vi "enable or disable module.vi"(6 "source":string, 7 "timeout":i32, 8 "error in (no error)":errorcluster, 9 "request type":T1, 10 "Module ID":string, 11 "Standard Engine Runtime in":refnum<class "Standard Engine Runtime.lvclass">) -> (0 "error out":errorcluster, 3 "Standard Engine Runtime out":refnum<class "Standard Engine Runtime.lvclass">)   [LabVIEW 2013, in "Standard Engine Runtime.lvclass"]
uses:
  Standard Engine Runtime.lvclass
  main engine/message request type.ctl
  main engine/message to engine.ctl
  global counter.vi
  main engine/main engine.lvlib
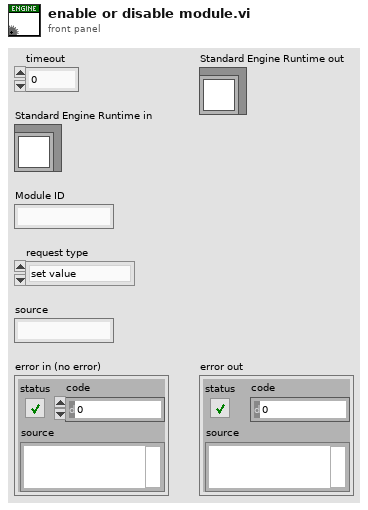
[diagram p1: front panel]
types:
  T1 = typedef "main engine.lvlib/message request type.ctl" = enum8{"set value", "disable module", "enable module"}
  T2 = typedef "main engine.lvlib/message to engine.ctl" = cluster{"request type":T1, "message ID":u8, "message field 1":u64, "message field 2":u64, "message field 3":u64, "message field 4":u64}
  T3 = typedef "main engine.lvlib/message from engine.ctl" = cluster{"response type":T4, "message ID":u8, "error code":i32}
  T4 = typedef "main engine.lvlib/message response type.ctl" = enum8{"ok", "error"}
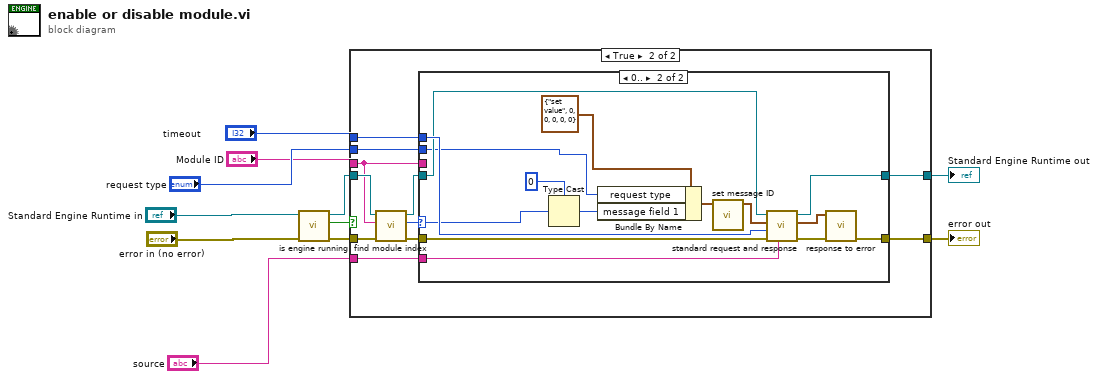
[diagram p0: block diagram]
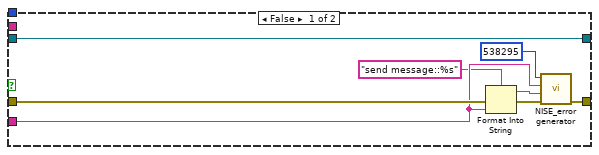
[diagram p2: hidden frame]
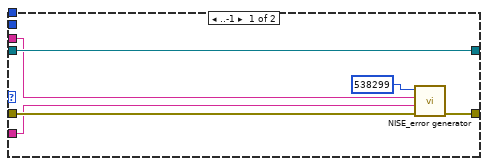
[diagram p3: hidden frame]
diagram:
  n1 = call "is engine running.vi"("error in"="error in (no error)", "Standard Engine Runtime in"="Standard Engine Runtime in") -> ("error out"=w7:errorcluster, "running?"=w3:bool, "Standard Engine Runtime out"=w5:refnum<class "Standard Engine Runtime.lvclass">)  [unwired: 7 in]
  n2 = case shown="True" w3 {
    tunnel: [w19 w30] -> w4
    tunnel: w5 -> [w19 w24]
    tunnel: [w17 w27] -> w6
    tunnel: w7 -> [w18 w26]
    tunnel: "timeout" -> [_ w28]
    tunnel: "source" -> [w14 w29]
    tunnel: "Module ID" -> [_ w21]
    tunnel: "request type" -> [_ w20]
    frame False {
      n3 = Format Into String(format string="send message::%s" ("source"), error in=w18, w14) -> (resulting string=w15:string, error out=w16:errorcluster)  [unwired: 1 in]
      n4 = call <vilib>:"NISE_error generator.vi"("error in"=w16, "source"=w15, "append error message"=w14, "error code (0)"=538295) -> ("error out"=w17:errorcluster)  [unwired: 5 in]
    }
    frame True {
      n5 = call "find module index.vi"("error in"=w26, "module ID"=w21, "Standard Engine Runtime in"=w24) -> ("error out"=w25:errorcluster, "index"=w22:i32, "Standard Engine Runtime out"=w23:refnum<class "Standard Engine Runtime.lvclass">)  [unwired: 6 in]
      n6 = case shown="0.." w22 {
        selector: w22 -> [_ w40]
        tunnel: [w35 w51] -> w30
        tunnel: w29 -> [w31 w50]
        tunnel: w28 -> [_ w49]
        tunnel: [w34 w47] -> w27
        tunnel: w25 -> [w36 w43]
        tunnel: w23 -> [w35 w42]
        tunnel: w21 -> [w32 _]
        tunnel: w20 -> [_ w37]
        frame ..-1 {
          n7 = call <vilib>:"NISE_error generator.vi"("error in"=w36, "source"=w31, "append error message"=w32, "error code (0)"=538299) -> ("error out"=w34:errorcluster)  [unwired: 5 in]
        }
        frame 0.. {
          n8 = Type Cast(type=u64 0, x=w40) -> (*(type *) &x=w39:u64)
          n9 = Bundle By Name(cluster=T2 {"request type"=enum."set value", "message ID"=0, "message field 1"=0, "message field 2"=0, "message field 3"=0, "message field 4"=0} ("request"), "request type"=w37, "message field 1"=w39) -> (w41:T2)
          n10 = call "set message ID.vi"("request in"=w41) -> ("request out"=w44:T2)  [unwired: 10 in]
          n11 = call "standard request and response.vi"("source if error"=w50, "error in"=w43, "timeout (-1)"=w49, "request"=w44, "Standard Engine Runtime in"=w42) -> ("error out"=w46:errorcluster, "message from engine"=w45:T3, "Standard Engine Runtime out"=w51:refnum<class "Standard Engine Runtime.lvclass">)  [unwired: 4 in]
          n12 = call "response to error.vi"("error in"=w46, "message from engine"=w45) -> ("error out"=w47:errorcluster)  [unwired: 9 in]
        }
      }
    }
  }
  "error out" <- w6
  "Standard Engine Runtime out" <- w4
